vi "Init 2 Talon Shooter With CVS Files.vi"(3 "error in":errorcluster, 4 "Shooter Right ID":string="Drive Right", 5 "Shooter Left ID":string="Drive Left", 6 "Robot ID":string="985") -> (0 "error out":errorcluster, 1 "Right PhoenixMotorControlDevRef":T1={"DeviceStatus"={"status"=FALSE, "code"=0, "source"=""}, "Type"=enum."PWM", "PWM"={"PWM Channel"=enum."PWM 1", "DeadBand"={"Name"="", "maxPositivePwm"=0, "minPositivePwm"=0, "centerPwm"=0, "maxNegativePwm"=0, "minNegativePwm"=0, "angularRange"=0}}, "CAN"={"Device Number"=0, "SetOutput VI Ref"=variant(enum8{"Percent VBus", "Current", "Speed", "Position", "Voltage"} enum."Percent VBus"), "GetOutput VI Ref"=variant(refnum<k1> refnum), "Enable VI Ref"=variant(dbl 12.0), "Disable VI Ref"=variant(enum8{"Percent VBus", "Speed", "Position", "Slave", "Unchanged / Invalid", "Voltage Compensation", "Current", "Motion Profile"} enum."Percent VBus"), "Data"=variant}, "Invert"=FALSE, "DIO PWM"={"PWM \"Enable\" Channel"=enum."Invalid", "DIOChannel"=enum."Invalid", "PWM Rate"=0.0}}, 2 "Left PhoenixMotorControlDevRef":T1={"DeviceStatus"={"status"=FALSE, "code"=0, "source"=""}, "Type"=enum."PWM", "PWM"={"PWM Channel"=enum."PWM 1", "DeadBand"={"Name"="", "maxPositivePwm"=0, "minPositivePwm"=0, "centerPwm"=0, "maxNegativePwm"=0, "minNegativePwm"=0, "angularRange"=0}}, "CAN"={"Device Number"=0, "SetOutput VI Ref"=variant(enum8{"Percent VBus", "Current", "Speed", "Position", "Voltage"} enum."Percent VBus"), "GetOutput VI Ref"=variant(refnum<k1> refnum), "Enable VI Ref"=variant(dbl 12.0), "Disable VI Ref"=variant(enum8{"Percent VBus", "Speed", "Position", "Slave", "Unchanged / Invalid", "Voltage Compensation", "Current", "Motion Profile"} enum."Percent VBus"), "Data"=variant}, "Invert"=FALSE, "DIO PWM"={"PWM \"Enable\" Channel"=enum."Invalid", "DIOChannel"=enum."Invalid", "PWM Rate"=0.0}})   [LabVIEW 2020]
uses:
  <vilib>/Rock Robotics/WPI/MotorControl/WPI_MotorControlDeviceRef.ctl
  <vilib>/Rock Robotics/WPI/MotorControl/WPI_MotorControlType.ctl
  <vilib>/Rock Robotics/SystemInterfaces/DIO/FPGA_DIOPWMChannel.ctl
  <vilib>/Rock Robotics/WPI/PWM/WPI_PWMDeadband.ctl
  <vilib>/Rock Robotics/SystemInterfaces/DIO/FPGA_DIOChannel.ctl
  <vilib>/Rock Robotics/WPI/SafetyOutput/WPI_SafetyOutputConfigMenu.ctl
  <vilib>/Rock Robotics/WPI/RobotDrive/WPI_RobotDriveOpen2MotorWithTalon.vi
panel:
  out "Shooter Right":u8
  out "Shooter Left":u8
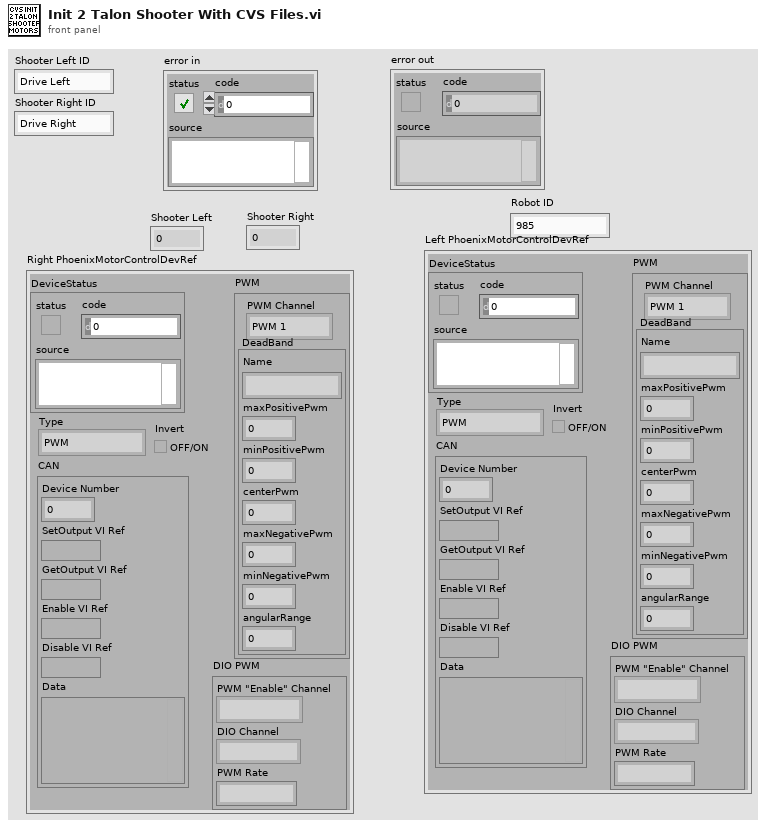
[diagram p1: front panel]
types:
  T1 = typedef "WPI_MotorControlDeviceRef.ctl" = cluster{"DeviceStatus":errorcluster, "Type":T2, "PWM":cluster{"PWM Channel":T3, "DeadBand":T4}, "CAN":cluster{"Device Number":u8, "SetOutput VI Ref":variant, "GetOutput VI Ref":variant, "Enable VI Ref":variant, "Disable VI Ref":variant, "Data":variant}, "Invert":bool, "DIO PWM":cluster{"PWM \"Enable\" Channel":T3, "DIOChannel":T5, "PWM Rate":dbl}}
  T2 = typedef "WPI_MotorControlType.ctl" = enum16{"PWM", "CAN", "DIO PWM"}
  T3 = typedef "FPGA_DIOPWMChannel.ctl" = enum8{"PWM 0", "PWM 1", "PWM 2", "PWM 3", "PWM 4", "PWM 5", "PWM 6", "PWM 7", "PWM 8", "PWM 9", "PWM MXP 0", "PWM MXP 1", "PWM MXP 2", "PWM MXP 3", "PWM MXP 4", "PWM MXP 5", "PWM MXP 6", "PWM MXP 7", "PWM MXP 8", "PWM MXP 9", "Invalid"}
  T4 = typedef "WPI_PWMDeadband.ctl" = cluster{"Name":string, "maxPositivePwm":i32, "minPositivePwm":i32, "centerPwm":i32, "maxNegativePwm":i32, "minNegativePwm":i32, "angularRange":u16}
  T5 = typedef "FPGA_DIOChannel.ctl" = enum8{"DIO 0", "DIO 1", "DIO 2", "DIO 3", "DIO 4", "DIO 5", "DIO 6", "DIO 7", "DIO 8", "DIO 9", "DIO MXP 0", "DIO MXP 1", "DIO MXP 2", "DIO MXP 3", "DIO MXP 4", "DIO MXP 5", "DIO MXP 6", "DIO MXP 7", "DIO MXP 8", "DIO MXP 9", "DIO MXP 10", "DIO MXP 11", "DIO MXP 12", "DIO MXP 13", "DIO MXP 14", "DIO MXP 15", "SPI Port CS1", "SPI Port CS2", "SPI Port CS3", "SPI Port MISO", "SPI Port MOSI", "Invalid"}
  T6 = typedef "WPI_SafetyOutputConfigMenu.ctl" = enum16{"Enable", "Disable"}
  T7 = typedef "WPI_RobotDriveDevRef.ctl" = cluster{"DevStatus":errorcluster, "Motors[]":T1[], "Square Inputs":bool, "Max Output":dbl}
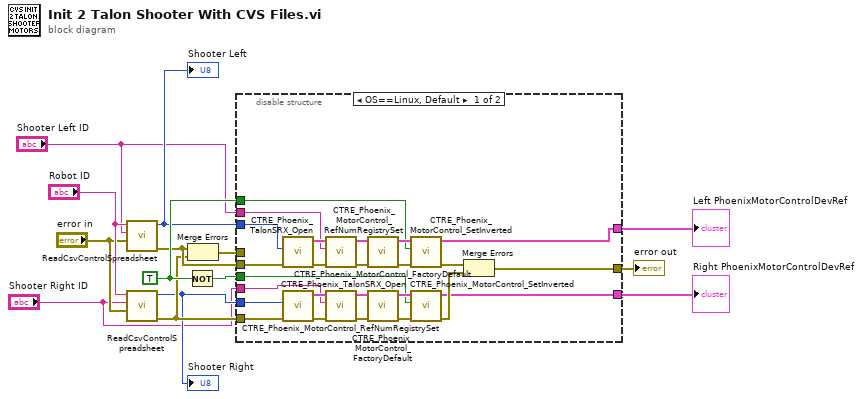
[diagram p0: block diagram]
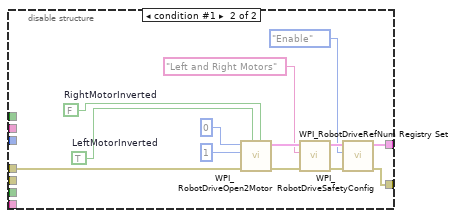
[diagram p2: hidden frame]
diagram:
  w13 = TRUE ("Invert")
  n1 = call "ReadCsvControlSpreadsheet.vi"("error in"="error in", "Motor ID"="Shooter Left ID", "Robot ID"="Robot ID") -> ("error out"=w9:errorcluster, "Can Bus ID"=w6:u8)  [unwired: 7 out]
  "Shooter Left" <- w6
  n2 = call "ReadCsvControlSpreadsheet.vi"("error in"="error in", "Motor ID"="Shooter Right ID", "Robot ID"="Robot ID") -> ("error out"=w8:errorcluster, "Can Bus ID"=w5:u8)  [unwired: 7 out]
  "Shooter Right" <- w5
  n3 = Not(x=w13) -> (.not. x?=w14:bool)
  n4 = Merge Errors(w9, w8) -> (w11:errorcluster)
  n5 = disable-structure shown="OS==Linux, Default" {
    disable-tunnel: w14 -> [w29 _]
    disable-tunnel: w13 -> [w32 _]
    disable-tunnel: w6 -> [w34 _]
    disable-tunnel: w5 -> [w31 _]
    disable-tunnel: [w28 w43] -> w4
    disable-tunnel: w11 -> [_ w42]
    disable-tunnel: [w27 w40] -> w10
    disable-tunnel: w9 -> [w33 _]
    disable-tunnel: w8 -> [w30 _]
    disable-tunnel: [w26 _] -> w3
    disable-tunnel: "Shooter Right ID" -> [w16 _]
    disable-tunnel: "Shooter Left ID" -> [w15 _]
    frame condition #0 (active) {
      n6 = call <vilib>:"CTRE_Phoenix_TalonSRX_Open.vi"("error in"=w33, "Device Number"=w34) -> ("error out"=w24:errorcluster, "PhoenixMotorControlDevRef"=w25:T1)  [unwired: 8 in]
      n7 = call <vilib>:"CTRE_Phoenix_TalonSRX_Open.vi"("error in"=w30, "Device Number"=w31) -> ("error out"=w20:errorcluster, "PhoenixMotorControlDevRef"=w21:T1)  [unwired: 8 in]
      n8 = call <vilib>:"CTRE_Phoenix_MotorControl_RefNumRegistrySet.vi"("error in (no error)"=w24, "refnum name"=w15, "PhoenixMotorControlDevRef"=w25) -> ("error out"=w22:errorcluster, "PhoenixMotorControlDevRef"=w23:T1)  [unwired: 7 in]
      n9 = call <vilib>:"CTRE_Phoenix_MotorControl_RefNumRegistrySet.vi"("error in (no error)"=w20, "refnum name"=w16, "PhoenixMotorControlDevRef"=w21) -> ("error out"=w17:errorcluster, "PhoenixMotorControlDevRef"=w18:T1)  [unwired: 7 in]
      n10 = call <vilib>:"CTRE_Phoenix_MotorControl_FactoryDefault.vi"("error in"=w22, "PhoenixMotorControlDevRef"=w23) -> ("error out"=w38:errorcluster, "PhoenixMotorControlDevRef"=w39:T1)  [unwired: 8 in]
      n11 = call <vilib>:"CTRE_Phoenix_MotorControl_FactoryDefault.vi"("error in"=w17, "PhoenixMotorControlDevRef"=w18) -> ("error out"=w19:errorcluster, "PhoenixMotorControlDevRef"=w37:T1)  [unwired: 8 in]
      n12 = call <vilib>:"CTRE_Phoenix_MotorControl_SetInverted.vi"("error in (no error)"=w38, "Invert?"=w32, "PhoenixMotorControlDevRef"=w39) -> ("error out"=w36:errorcluster, "PhoenixMotorControlDevRef"=w28:T1)  [unwired: 7 in]
      n13 = call <vilib>:"CTRE_Phoenix_MotorControl_SetInverted.vi"("error in (no error)"=w19, "Invert?"=w29, "PhoenixMotorControlDevRef"=w37) -> ("error out"=w35:errorcluster, "PhoenixMotorControlDevRef"=w26:T1)  [unwired: 7 in]
      n14 = Merge Errors(w36, w35) -> (w27:errorcluster)
    }
    frame condition #1 {
      w47 = TRUE  # LeftMotorInverted
      w48 = FALSE  # RightMotorInverted
      n15 = call-poly <vilib>:"WPI_RobotDriveOpen2Motor.vi"("Right Motor Inverted"=w48, "Left Motor Inverted"=w47, "error in (no error)"=w42, "Right Motor"=u8 1 ("Left Motor"), "Left Motor"=u8 0) -> ("error out"=w51:errorcluster, "RobotDriveDevRef"=w50:T7)  [unwired: 5 out]
      n16 = call <vilib>:"WPI_RobotDriveRefNum Registry Set.vi"("error in (no error)"=w51, "refnum name"="Left and Right Motors", "RobotDriveDevRef"=w50) -> ("error out"=w41:errorcluster, "RobotDriveDevRef"=w52:T7)  [unwired: 1 in, 6 out]
      n17 = call <vilib>:"WPI_RobotDriveSafetyConfig.vi"("error in (no error)"=w41, "mode"=WPI_SafetyOutputConfigMenu."Enable", "RobotDriveDevRef"=w52) -> ("error out"=w40:errorcluster, "RobotDriveDevRef"=w43:T7)  [unwired: 7 in]
    }
  }
  "error out" <- w10
  "Left PhoenixMotorControlDevRef" <- w4
  "Right PhoenixMotorControlDevRef" <- w3
